vi "Initialization.vi"(8 "error in (no error)":errorcluster, 11 "Prooduct Actor in":refnum<class "Prooduct Actor.lvclass">) -> (0 "error out":errorcluster, 3 "Prooduct Actor out":refnum<class "Prooduct Actor.lvclass">)   [LabVIEW 2020, in "Prooduct Actor.lvlib" / "Prooduct Actor.lvclass"]
uses:
  Prooduct Actor.lvclass
  Prooduct Actor.lvclass/Prooduct Actor.ctl
  Read Product Sub Panel.vi
  Read VI Refnum.vi
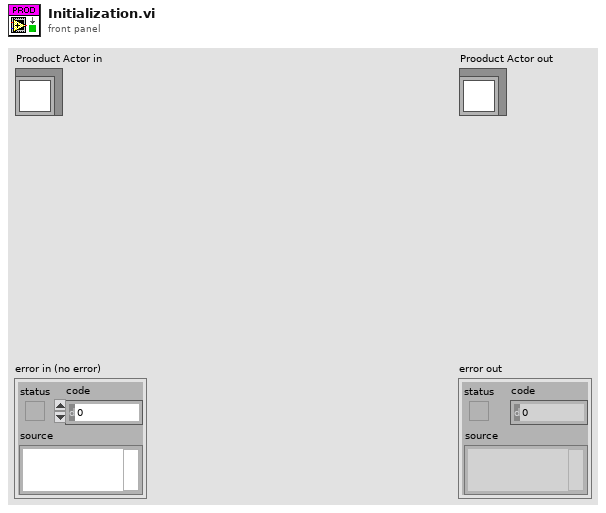
[diagram p1: front panel]
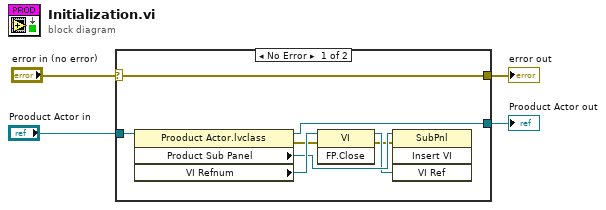
[diagram p0: block diagram]
diagram:
  n1 = case shown="No Error" "error in (no error)" {
    selector: "error in (no error)" -> [w11 w14]
    tunnel: [w11 w14] -> w3
    tunnel: [w10 w13] -> w1
    tunnel: "Prooduct Actor in" -> [w12 w13]
    frame No Error {
      n2 = property class="Prooduct Actor.lvclass"(reference=w12) -> (reference out=w10:refnum<class "Prooduct Actor.lvclass">, error out=w5:errorcluster, "Product Sub Panel"=w8:refnum<vi>, "VI Refnum"=w9:refnum<vi>)  [unwired: 1 in]
      n3 = invoke class="VI" method="FP.Close"(reference=w9, error in=w5) -> (reference out=w7:refnum<vi>, error out=w6:errorcluster)  [unwired: 1 in, 1 out]
      n4 = invoke class="SubPnl" method="Insert VI"(reference=w8, error in=w6, "VI Ref"=w7) -> ()  [unwired: 1 in, 4 out]
    }
    frame Error {
    }
  }
  "error out" <- w3
  "Prooduct Actor out" <- w1
